vi "FTW-TestExecutive-Core_StepTypes_Set.vi"(0 "FTW-TestExecutive-Core In":refnum<class "FTW-TestExecutive-Core.lvclass">, 7 "Step Types":cluster{"Name":string, "Base Config":string}[](array[cluster]), 11 "error in":errorcluster) -> (4 "FTW-TestExecutive-Core Out":refnum<class "FTW-TestExecutive-Core.lvclass">, 15 "error out":errorcluster)   [LabVIEW 2015, in "FTW-TestExecutive-Core.lvclass"]
uses:
  FTW-TestExecutive-Core.lvclass
  FTW-TestExecutive-Core.lvclass/FTW-TestExecutive-Core.ctl
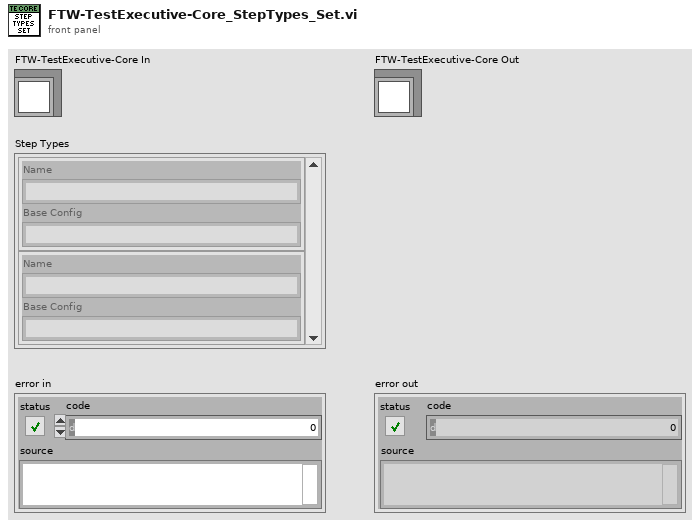
[diagram p1: front panel]
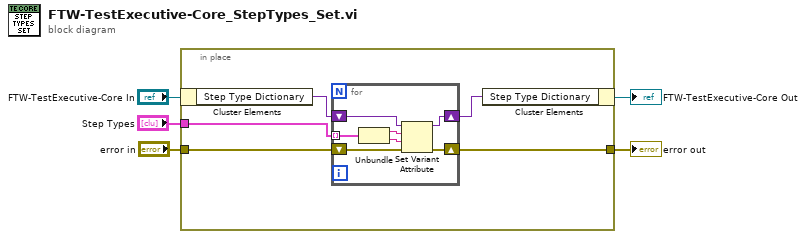
[diagram p0: block diagram]
diagram:
  n1 = in-place {
    in-place-border: "Step Types" -> [w8]
    in-place-border: "error in" -> [w7]
    in-place-border: [w6] -> w3
    n2 = in-place-cluster #1("FTW-TestExecutive-Core In") -> ("Step Type Dictionary"=w10:variant)
    n3 = for {
      shift-right: [w16] -> w6
      shift-left: w7 -> [w17]
      shift-right: [w14] -> w9
      shift-left: w10 -> [w15]
      tunnel: w8 -> [w13] mode=indexing
      n4 = Unbundle(w13) -> ("Name"=w12:string, "Base Config"=w11:string)
      n5 = Set Variant Attribute(Variant=w15, name=w12, value=w11, error in=w17) -> (Variant out=w14:variant, error out=w16:errorcluster)  [unwired: 1 out]
    }
    n6 = in-place-cluster #1("Step Type Dictionary"=w9) -> (→"FTW-TestExecutive-Core Out":refnum<class "FTW-TestExecutive-Core.lvclass">)
  }
  "error out" <- w3
